vi "Write Text.vi"(8 "error in (no error)":errorcluster, 10 "Text":string, 11 "MGI_MenuItem in":refnum<class "MGI_MenuItem.lvclass">) -> (0 "error out":errorcluster, 3 "MGI_MenuItem out":refnum<class "MGI_MenuItem.lvclass">)   [LabVIEW 2016, in "MGI_MenuItem.lvclass"]
doc: "This is the text displayed to the user.\n\nAuthored by Derek E. Trepanier\nsupport@mooregoodideas.com\nwww.mooregoodideas.com\n\nCopyright (c) 2012, Moore Good Ideas, Inc.\n\nAll rights reserved.\n\nRedistribution and use in source and binary forms, with or without modification, are permitted provided that the following conditions are met:\n\n * Redistributions of source code must retain the above copyright notice, this list of conditions and the following disclaimer.\n * Redistributions in binary form must reproduce the above copyright notice, this list of conditions and the following disclaimer in the documentation and/or other materials provided with the distribution.\n * Neither the name of Moore Good Ideas, Inc. nor the names of its contributors may be used to endorse or promote products derived from this software without specific prior written permission.\n\nTHIS SOFTWARE IS PROVIDED BY THE COPYRIGHT HOLDERS AND CONTRIBUTORS \"AS IS\" AND ANY EXPRESS OR IMPLIED WARRANTIES, INCLUDING, BUT NOT LIMITED TO, THE IMPLIED WARRANTIES OF MERCHANTABILITY AND FITNESS FOR A PARTICULAR PURPOSE ARE DISCLAIMED. IN NO EVENT SHALL THE COPYRIGHT OWNER OR CONTRIBUTORS BE LIABLE FOR ANY DIRECT, INDIRECT, INCIDENTAL, SPECIAL, EXEMPLARY, OR CONSEQUENTIAL DAMAGES (INCLUDING, BUT NOT LIMITED TO, PROCUREMENT OF SUBSTITUTE GOODS OR SERVICES; LOSS OF USE, DATA, OR PROFITS; OR BUSINESS INTERRUPTION) HOWEVER CAUSED AND ON ANY THEORY OF LIABILITY, WHETHER IN CONTRACT, STRICT LIABILITY, OR TORT (INCLUDING NEGLIGENCE OR OTHERWISE) ARISING IN ANY WAY OUT OF THE USE OF THIS SOFTWARE, EVEN IF ADVISED OF THE POSSIBILITY OF SUCH DAMAGE."
uses:
  <userlib>/_MGI/Menu Building/MenuItem/MGI_MenuItem.lvclass
  <userlib>/_MGI/Menu Building/MenuItem/MGI_MenuItem.lvclass/MGI_MenuItem.ctl
  <userlib>/_MGI/Menu Building/MenuItem/Write Tag.vi
  <userlib>/_MGI/Menu Building/MenuTypes/MGI_Menu.lvclass
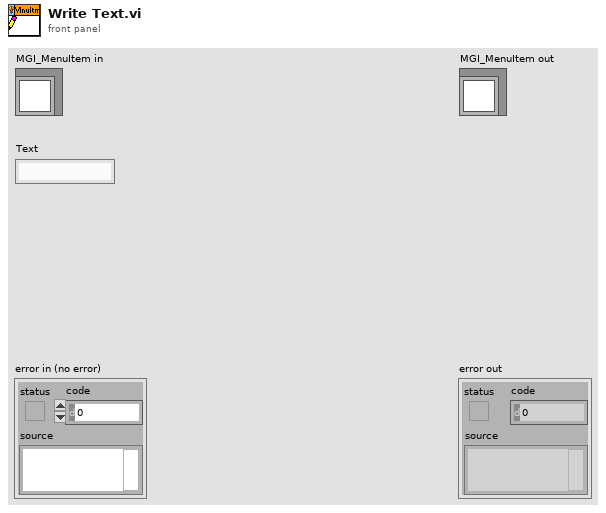
[diagram p1: front panel]
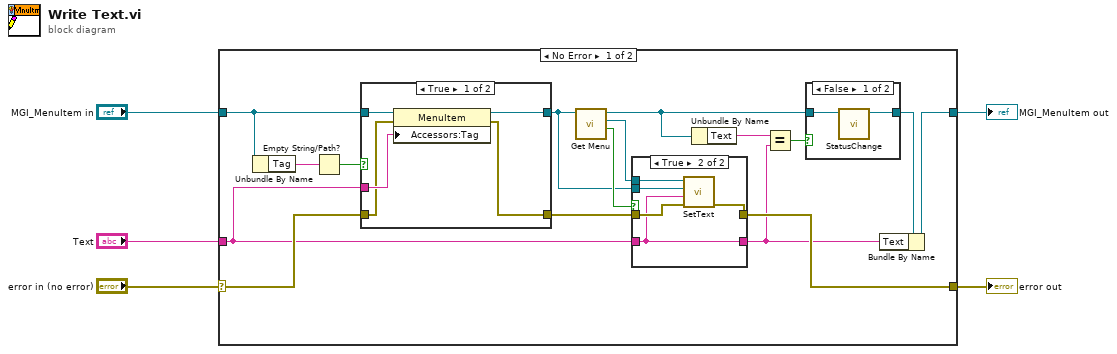
[diagram p0: block diagram]
diagram:
  n1 = case shown="No Error" "error in (no error)" {
    selector: "error in (no error)" -> [w18 w39]
    tunnel: [w13 w39] -> w4
    tunnel: [w11 w40] -> w2
    tunnel: "MGI_MenuItem in" -> [w21 w40]
    tunnel: "Text" -> [w12 _]
    frame No Error {
      n2 = Unbundle By Name(w21) -> ("Tag"=w20:string)
      n3 = Empty String/Path?(string/path=w20) -> (empty?=w19:bool)
      n4 = case shown="True" w19 {
        tunnel: [w32 w38] -> w15
        tunnel: w12 -> [w35 _]
        tunnel: w21 -> [w36 w38]
        tunnel: w18 -> [w34 w37]
        tunnel: [w33 w37] -> w14
        frame True {
          n5 = property class="MenuItem"(reference=w36, error in=w34, "Accessors:Tag"=w35) -> (reference out=w32:refnum<class "MGI_MenuItem.lvclass">, error out=w33:errorcluster)
        }
        frame False {
        }
      }
      n6 = call <userlib>:"Get Menu.vi"("MenuItem in"=w15) -> ("Menu Valid"=w16:bool, "Menu"=w17:refnum<class "MGI_Menu.lvclass">, "MenuItem out"=w7:refnum<class "MGI_MenuItem.lvclass">)  [unwired: 7 in, 1 out]
      n7 = case shown="True" w16 {
        tunnel: w17 -> [_ w31]
        tunnel: w15 -> [_ w30]
        tunnel: w12 -> [w25 w27]
        tunnel: w14 -> [w26 w29]
        tunnel: [w26 w28] -> w13
        tunnel: [w25 w27] -> w8
        frame False {
        }
        frame True {
          n8 = call-dynamic "SetText.vi"("error in (no error)"=w29, "New Text"=w27, "MenuItem"=w30, "Menu in"=w31) -> ("error out"=w28:errorcluster)  [unwired: 6 in, 1 out]
        }
      }
      n9 = Unbundle By Name(w7) -> ("Text"=w6:string)
      n10 = Equal?(x=w6, y=w8) -> (x = y?=w9:bool)
      n11 = case shown="False" w9 {
        tunnel: w7 -> [w23 w24]
        tunnel: [w22 w24] -> w10
        frame False {
          n12 = call-dynamic "StatusChange.vi"("MGI_MenuItem in"=w23) -> ("MGI_MenuItem out"=w22:refnum<class "MGI_MenuItem.lvclass">)  [unwired: 9 in, 1 out]
        }
        frame True {
        }
      }
      n13 = Bundle By Name(cluster=w10, "Text"=w8) -> (w11:refnum<class "MGI_MenuItem.lvclass">)
    }
    frame Error {
    }
  }
  "error out" <- w4
  "MGI_MenuItem out" <- w2
